vi "Application Directory 2.vi"(4 "Relative path (.)":path=path "") -> (1 "Application Directory (+ Relative)":path)   [LabVIEW 2017]
doc: "Returns the application directory with Relative path (.) appended. An empty relative path returns the application directory itself."
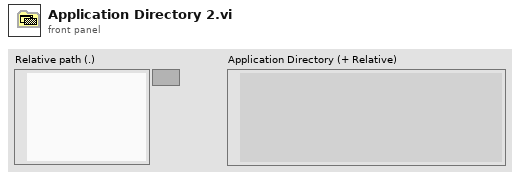
[diagram p1: front panel]
types:
  T1 = enum16{"Absolute path", "Relative path", "<Not A Path>"}
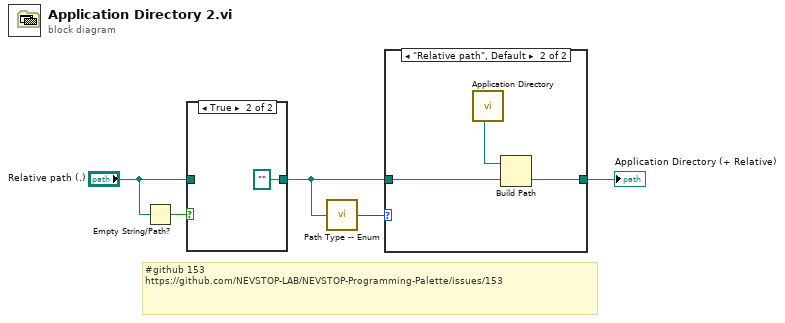
[diagram p0: block diagram]
diagram:
  # "#github 153\nhttps://github.com/NEVSTOP-LAB/NEVSTOP-Programming-Palette/issues/153"
  n1 = Empty String/Path?(string/path="Relative path (.)") -> (empty?=w3:bool)
  n2 = case shown="True" w3 {
    tunnel: [w6 path "" ("Relative path (.)")] -> w2
    tunnel: "Relative path (.)" -> [w6 _]
    frame False {
    }
    frame True {
    }
  }
  n3 = call "Path Type -- Enum.vi"("Value"=w2) -> ("Enum"=w4:T1)
  n4 = case shown="\"Relative path\", Default" w4 {
    tunnel: [w8 w11] -> w5
    tunnel: w2 -> [w8 w9]
    frame "Absolute path" {
    }
    frame "Relative path", Default {
      n5 = call <vilib>:"Application Directory.vi"() -> ("Application Directory"=w10:path)
      n6 = Build Path(base path=w10, name or relative path=w9) -> (appended path=w11:path)
    }
  }
  "Application Directory (+ Relative)" <- w5
